vi "visualizer.vi"(11 "Name (\"\" to Use UUID)":string="ui") -> ()   [LabVIEW 2025]
uses:
  acccbc90-5136-4eb0-8ada-bd77d99bf855.vi
  <userlib>/_NEVSTOP/Communicable State Machine(CSM)/AdvanceAPI/CSM - Revert Arguments-Safe String.vi
  <userlib>/_NEVSTOP/Communicable State Machine(CSM)/AdvanceAPI/CSM - Make String Arguments Safe.vi
  <userlib>/_NEVSTOP/Communicable State Machine(CSM)/AdvanceAPI/CSM - Break Down Multiple States String.vi
  <userlib>/_NEVSTOP/Communicable State Machine(CSM)/AdvanceAPI/CSM - Compact Multiple States.vi
  <userlib>/_NEVSTOP/Communicable State Machine(CSM)/AdvanceAPI/CSM - Keywords.vi
  <userlib>/_NEVSTOP/Communicable State Machine(CSM)/_Shared/Trim Single-line Text.vi
  <userlib>/_NEVSTOP/Communicable State Machine(CSM)/addons/MassData-Parameter/_support/FGV-MassData(lvlibp).vi
  <userlib>/_NEVSTOP/Communicable State Machine(CSM)/_Polymophic/Build Asynchronous Message with Arguments.vi
  <userlib>/_NEVSTOP/Communicable State Machine(CSM)/Communicable State Machine.lvlib
panel:
  out "Error Occurred":errorcluster
  out "State History":string
  in  "Exit":bool
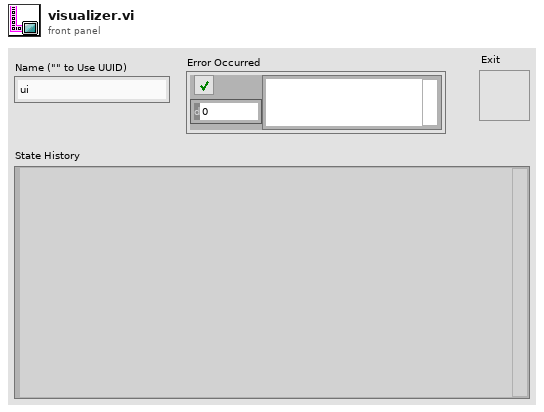
[diagram p1: front panel]
types:
  T1 = enum32{"Invalid", "Standard", "Closed", "Hidden", "Minimized", "Maximized"}
  T2 = enum32{"invalid app kind", "Development System", "Run Time System", "Student Edition", "Embedded LabVIEW", "Evaluation", "Custom"}
  T3 = typedef "Communicable State Machine.lvlib/_CSM_Response Source Message.ctl" = cluster{"‘State":string, "’Arguments":string, "’Error":errorcluster}
  T4 = cluster{"Current VI Reference":refnum<vi>, "Close Panel on Exit?":bool}
  T5 = cluster{"Core":cluster{"Current VI Reference":refnum<vi>, "Close Panel on Exit?":bool}, "rect":cluster{"left":i16, "top":i16, "right":i16, "bottom":i16}}
  T6 = cluster{"left":i16, "top":i16, "right":i16, "bottom":i16}
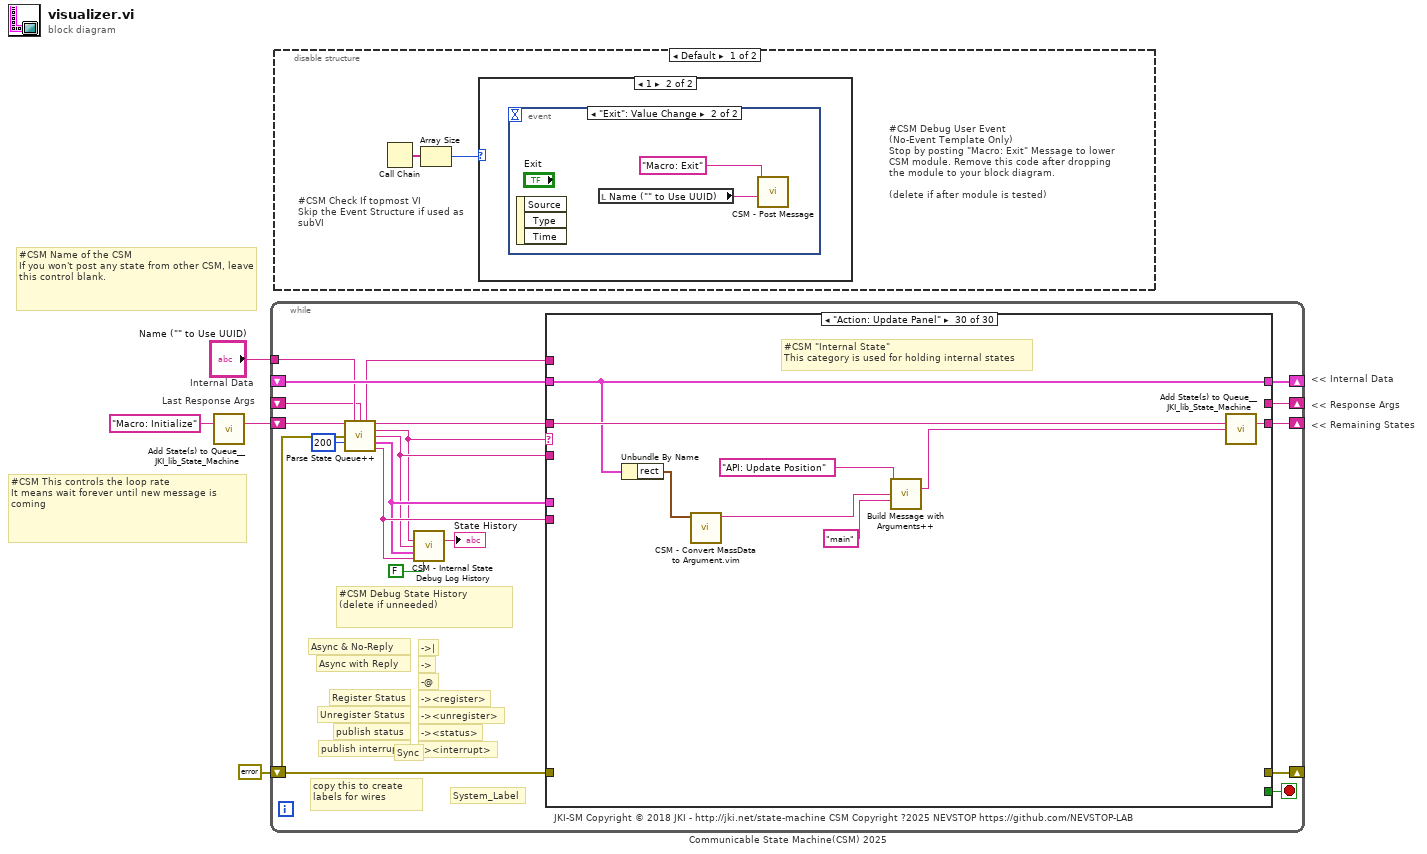
[diagram p0: block diagram]
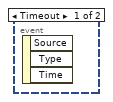
[diagram p3: hidden frame]
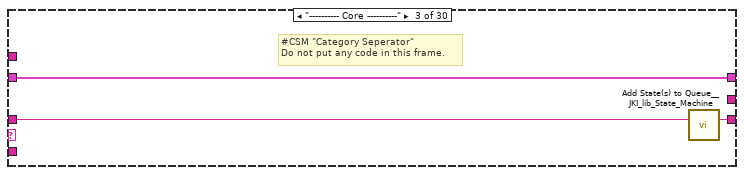
[diagram p7: hidden frame]
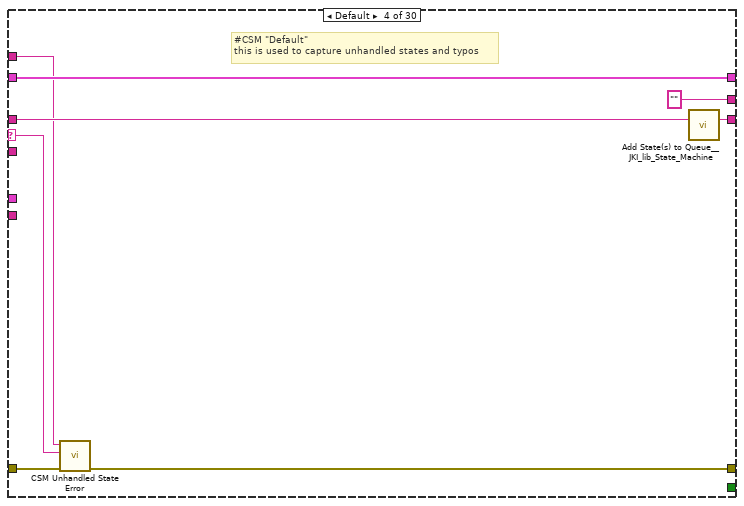
[diagram p8: hidden frame]
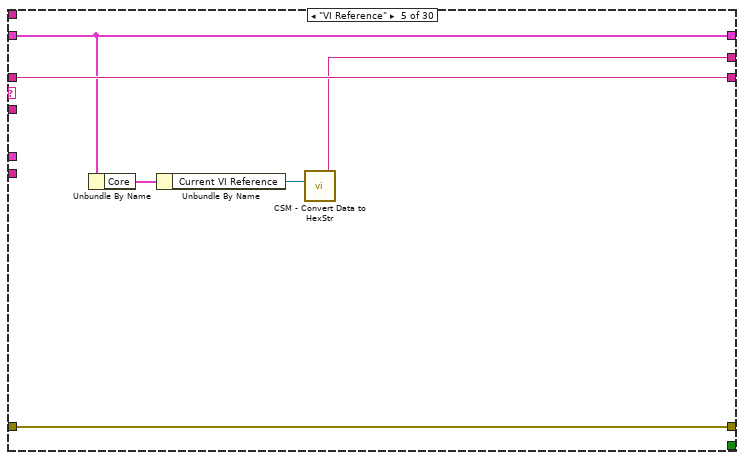
[diagram p9: hidden frame]
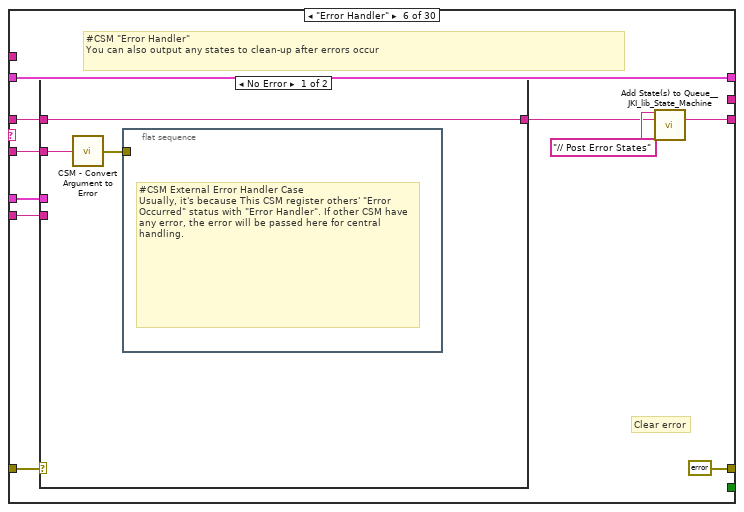
[diagram p10: hidden frame]
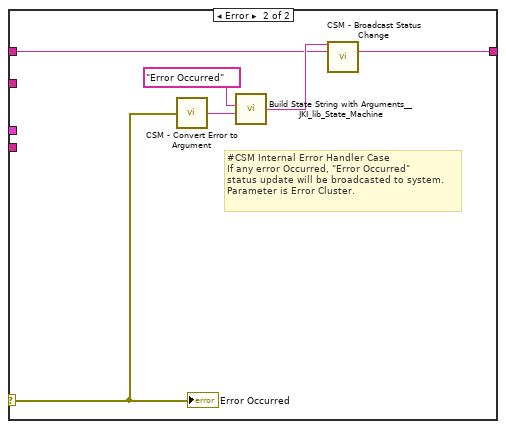
[diagram p11: hidden frame]
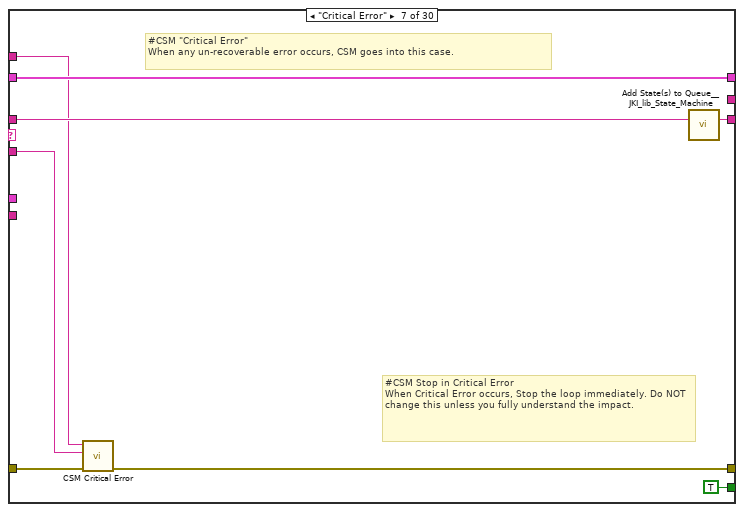
[diagram p12: hidden frame]
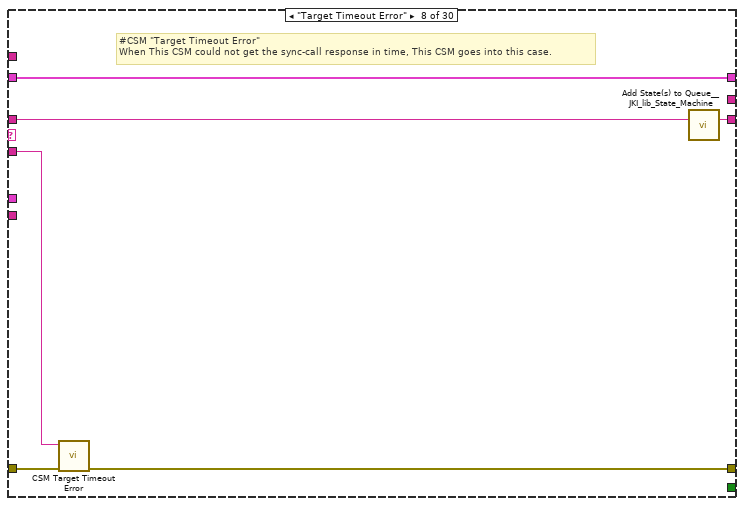
[diagram p13: hidden frame]
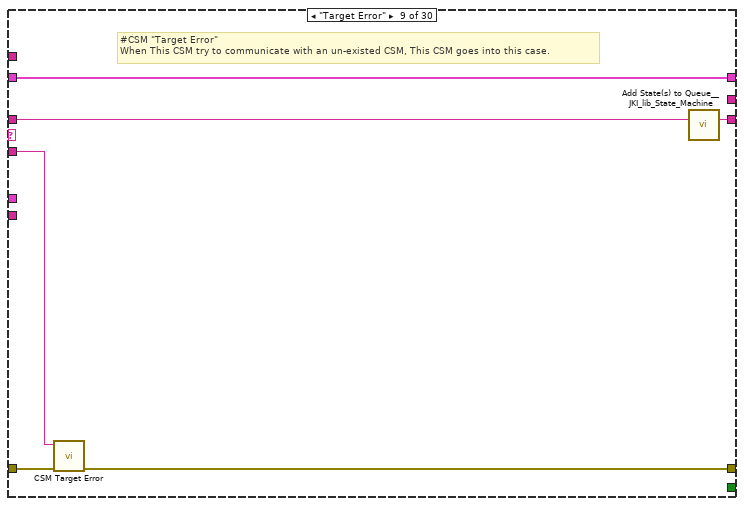
[diagram p14: hidden frame]
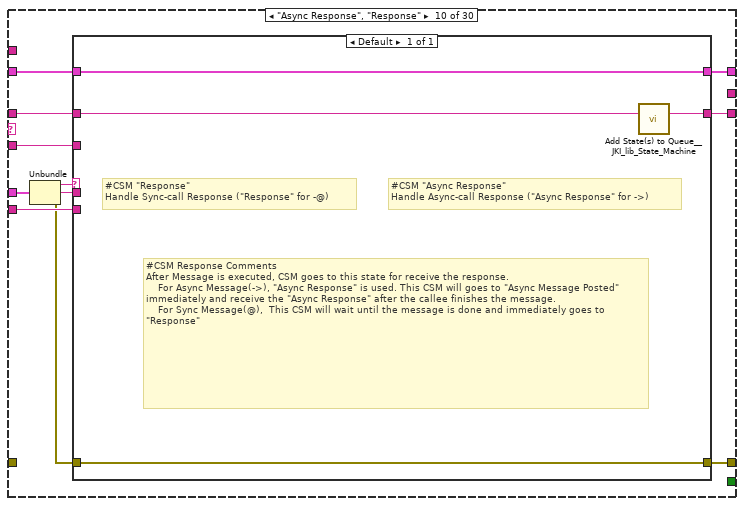
[diagram p15: hidden frame]
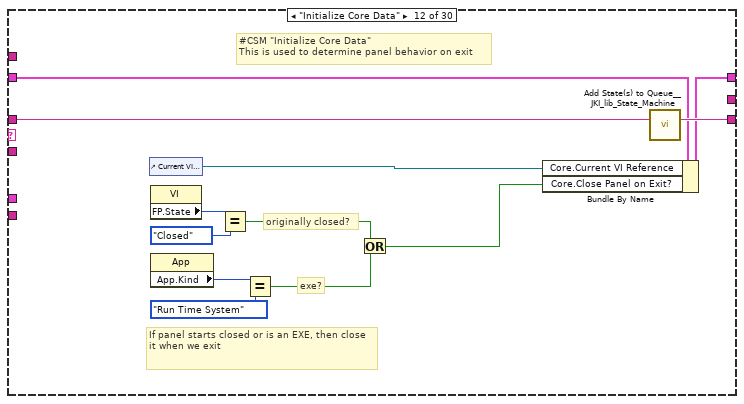
[diagram p17: hidden frame]
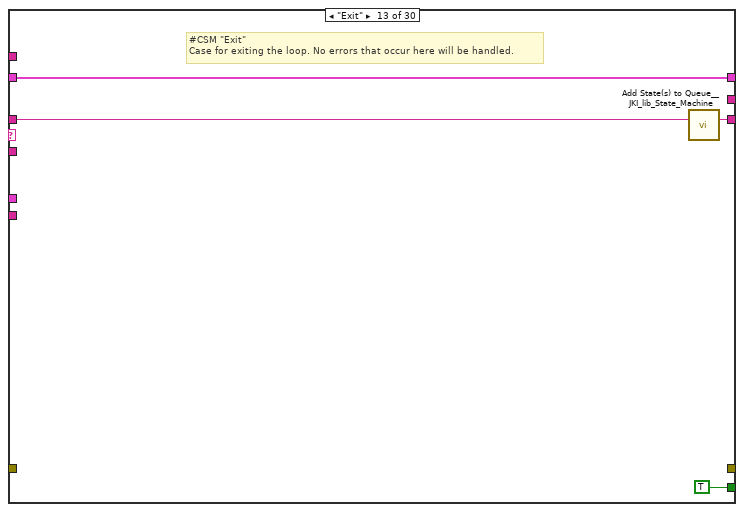
[diagram p18: hidden frame]
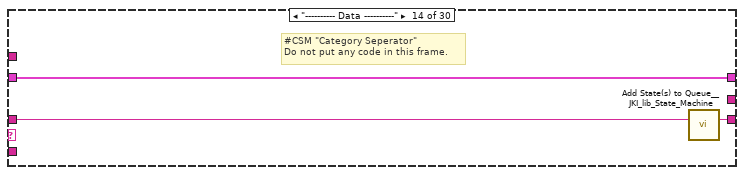
[diagram p19: hidden frame]
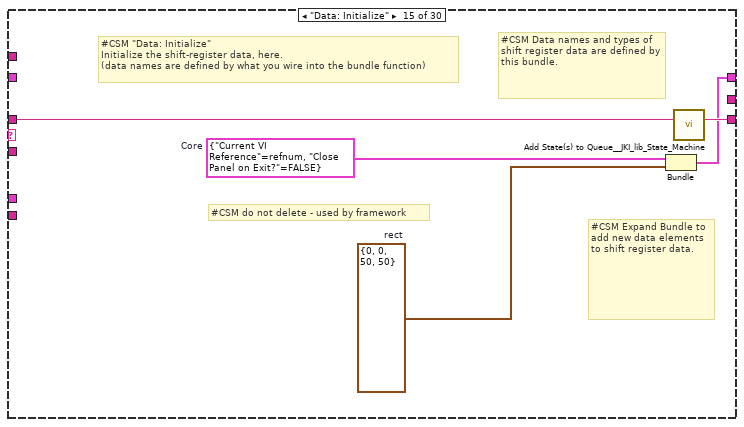
[diagram p20: hidden frame]
diagram:
  # "Last Response Args"
  # "Internal Data"
  # "#CSM Name of the CSM\nIf you won't post any state from other CSM, leave this control blank."
  # "#CSM This controls the loop rate\nIt means wait forever until new message is coming"
  # "<< Internal Data"
  # "<< Response Args"
  # "<< Remaining States"
  n1 = call <vilib>:"Add State(s) to Queue__JKI_lib_State_Machine.vi"("State(s) in (\"\")"="Macro: Initialize" ("Init State(\"Macro: Initialize\")")) -> ("States Out"=w1:string)  [unwired: 14 in]
  n2 = while "Communicable State Machine(CSM) 2025" {
    shift-right: [w18] -> _
    shift-left: _ -> [w17]
    shift-right: [w21] -> _
    shift-left: errorcluster {"status"=FALSE, "code"=0, "source"=""} ("error out") -> [w8]
    shift-right: [w20] -> _
    shift-left: w1 -> [w22]
    tunnel: "Name (\"\" to Use UUID)" -> [w15]
    shift-right: [w16] -> _
    shift-left: _ -> [w10]
    stop <- w19 stop-if-true
    # "#CSM Debug State History\n(delete if unneeded)"
    # "-><interrupt>"
    # "-><status>"
    # "-><unregister>"
    # "-><register>"
    # "-@"
    # "->"
    # "->|"
    # "publish interrupt"
    # "publish status"
    # "Unregister Status"
    # "Register Status"
    # "Sync"
    # "Async with Reply"
    # "Async & No-Reply"
    # "JKI-SM Copyright © 2018 JKI - http://jki.net/state-machine CSM Copyright ?2025 NEVSTOP https://github.com/NEVSTOP-LAB"
    # "copy this to create labels for wires"
    # "System_Label"
    n3 = call <userlib>:"Parse State Queue++.vi"("State Queue"=w22, "Name (\"\" to Use UUID)"=w15, "Response Arguments"=w10, "Previous Error"=w8, "Dequeue (1 ms)"=200) -> ("Name Used"=w9:string, "Remaining States"=w23:string, "Current State"=w11:string, "Arguments"=w12:string, "Additional Information"=w13:T3, "Source CSM"=w14:string)  [unwired: 5 in]
    n4 = call <userlib>:"CSM - Internal State Debug Log History.vi"("State"=w11, "Arguments (\"\")"=w12, ">> Response Source Message >>"=w13, "Source (\"\")"=w14, "Enable Periodic State Filter? (T)"=FALSE) -> ("Debug Log"=→"State History":string)  [unwired: 10 in]
    n5 = case shown="\"Action: Update Panel\"" w11 {
      selector: w11 -> [_ _ _ w34 _ _ _ _ _ _ _ _ _ _ _ _ _ _ _ _ _ _ _ _ _ _ _ _ _ _]
      tunnel: w23 -> [w24 w27 w30 w38 w43 w48 w71 w77 w83 w93 w100 w112 w116 w119 w124 w126 w132 w135 w139 w145 w147 w150 w153 w156 w166 w177 w188 w199 w203 w211]
      tunnel: w12 -> [_ _ _ _ _ w47 w67 w74 w80 w87 _ _ _ _ _ _ _ _ _ _ _ _ _ _ _ _ _ _ _ _]
      tunnel: w17 -> [w25 w26 w28 w36 w42 w53 w69 w75 w81 w91 w99 w106 w114 w117 _ w125 w127 w133 w137 w143 w146 w149 w152 w155 w160 w171 w182 w193 w201 w207]
      tunnel: [_ _ _ w31 w44 errorcluster {"status"=FALSE, "code"=0, "source"=""} ("error out") w64 w72 w78 w94 _ _ _ _ _ _ w128 _ _ _ w148 w151 w154 _ _ _ _ _ _ _] -> w21
      tunnel: w8 -> [_ _ _ w32 w44 w51 w65 w73 w79 _ _ _ _ _ _ _ w129 _ _ _ w148 w151 w154 _ _ _ _ _ _ _]
      tunnel: [w24 w27 w29 w37 w43 w49 w70 w76 w82 w92 w100 w111 w115 w118 w123 w126 w131 w134 w138 w144 w147 w150 w153 w156 w165 w176 w187 w198 w202 w210] -> w20
      tunnel: [_ _ _ _ _ _ TRUE _ _ _ _ _ TRUE _ _ _ _ _ _ _ _ _ _ _ _ _ _ _ _ _] -> w19
      tunnel: [w25 w26 w28 w36 w42 w53 w69 w75 w81 w90 w99 w110 w114 w117 w122 w125 w127 w133 w137 w143 w146 w149 w152 w155 w159 w170 w181 w192 w201 w207] -> w18
      tunnel: w14 -> [_ _ _ _ _ w46 _ _ _ w88 _ _ _ _ _ _ _ _ _ _ _ _ _ _ _ _ _ _ _ _]
      tunnel: w13 -> [_ _ _ _ _ w45 _ _ _ w89 _ _ _ _ _ _ _ _ _ _ _ _ _ _ _ _ _ _ _ _]
      tunnel: [_ _ _ "" w39 _ _ _ _ _ _ _ _ _ _ _ _ _ _ _ _ _ _ _ "Moved Up" ("HEX String (0-9,A-F)") "Moved Up" ("HEX String (0-9,A-F)") "Moved Up" ("HEX String (0-9,A-F)") "Moved Up" ("HEX String (0-9,A-F)") _ _] -> w16
      tunnel: w9 -> [_ _ _ w33 _ _ w66 _ _ _ _ _ _ _ _ _ _ _ _ _ _ _ _ _ _ _ _ _ _ _]
      frame "", "Idle" {
        # "#CSM \"Idle/Event Handler\"\nexecutes when the state queue is empty"
      }
      frame "CSM Documentation" {
        # "#CSM State Syntax\n\n// Comment line, all text to the right of “//” will be ignored\n// Local Message Example\nDoSth: DoA >> Arguments\n\n// Sync Call Example\nAPI: xxxx >> Arguments -@ TargetModule\n\n// Async Call Example\nAPI: xxxx >> Arguments -> TargetModule\n\n// Async Call without Reply Example\nAPI: xxxx >> Arguments ->| TargetModule\n\n// Broadcast normal status:\nStatus >> StatusArguments  -><status>\n\n// Broadcast Interrupt status:\nInterrupt >> StatusArguments  -><interrupt>\n\n// Register Source Module's status to Handler Module\nStatus@Source Module >> Handler Module@Handler Module -><register>\n\n// Unegister Source Module's status\nStatus@Source Module >> Handler Module -><unregister>"
        # "#CSM README FIRST\n\nCommunicable State Machine(CSM) is a LabVIEW application framework that builds upon JKI State Machine(JKISM). It follows the pattern of JKISM and extends the keywords to describe message communication between modules, including concepts such as Sync-Message, Async-Message, Subscription/Unsubscription of status - essential elements for creating reusable code modules. For more information, please visit the CSM wiki: https://nevstop-lab.github.io/CSM-Wiki/\n\nFor instructions on JKI State Machine, visit: \n    http://jki.net/state-machine/\nFor information about CSM, visit: \n    https://github.com/NEVSTOP-LAB"
        # "#CSM \"Documentation\"\nCase for holding CSM Documenation"
      }
      frame "---------- Core ----------" {
        # "#CSM \"Category Seperator\"\nDo not put any code in this frame."
        n6 = call <vilib>:"Add State(s) to Queue__JKI_lib_State_Machine.vi"("State(s) in (\"\")"=w30) -> ("States Out"=w29:string)  [unwired: 14 in]
      }
      frame Default {
        # "#CSM \"Default\"\nthis is used to capture unhandled states and typos"
        n7 = call <userlib>:"CSM Unhandled State Error.vi"("error in (no error)"=w32, "Undefined State"=w34, "CSM Name"=w33) -> ("error out"=w31:errorcluster)  [unwired: 8 in]
        n8 = call <vilib>:"Add State(s) to Queue__JKI_lib_State_Machine.vi"("State(s) in (\"\")"=w38) -> ("States Out"=w37:string)  [unwired: 14 in]
      }
      frame "VI Reference" {
        n9 = Unbundle By Name(w42) -> ("Core"=w41:T4)
        n10 = Unbundle By Name(w41) -> ("Current VI Reference"=w40:refnum<vi>)
        n11 = call <userlib>:"CSM - Convert Data to HexStr.vi"("Variant"=w40) -> ("HEX String (0-9,A-F)"=w39:string)  [unwired: 8 in]
      }
      frame "Error Handler" {
        # "#CSM \"Error Handler\"\nYou can also output any states to clean-up after errors occur"
        # "Clear error"
        n12 = case shown="No Error" w51 {
          selector: w51 -> [_ w58]
          tunnel: [w57 w60] -> w50
          tunnel: w48 -> [w57 w59]
          tunnel: w47 -> [w56 _]
          tunnel: w46 -> [_ _]
          tunnel: w45 -> [_ _]
          frame No Error {
            n13 = call <userlib>:"CSM - Convert Argument to Error.vi"("Argument"=w56) -> ("Error"=w55:errorcluster)  [unwired: 4 in]
            n14 = flat-sequence {
              tunnel: w55 -> [_]
              frame #0 {
                # "#CSM External Error Handler Case\nUsually, it's because This CSM register others' \"Error Occurred\" status with \"Error Handler\". If other CSM have any error, the error will be passed here for central handling."
              }
            }
          }
          frame Error {
            # "#CSM Internal Error Handler Case \nIf any error Occurred, \"Error Occurred\" \nstatus update will be broadcasted to system.\nParameter is Error Cluster."
            n15 = call <userlib>:"CSM - Convert Error to Argument.vi"("Error"=w58) -> ("Argument"=w62:string)  [unwired: 4 in]
            n16 = call <vilib>:"Build State String with Arguments__JKI_lib_State_Machine.vi"("Arguments (\"\")"=w62, "State"="Error Occurred" ("Status with Arguments")) -> ("State with Arguments"=w61:string)  [unwired: 4 in]
            n17 = call <userlib>:"CSM - Broadcast Status Change.vi"("Status With Arguments"=w61, "State Queue"=w59) -> ("Remaining States"=w60:string)  [unwired: 13 in]
            "Error Occurred" <- w58
          }
        }
        n18 = call <vilib>:"Add State(s) to Queue__JKI_lib_State_Machine.vi"("State(s) in Front (\"\")"="// Post Error States", "State(s) in (\"\")"=w50) -> ("States Out"=w49:string)  [unwired: 13 in]
      }
      frame "Critical Error" {
        # "#CSM \"Critical Error\"\nWhen any un-recoverable error occurs, CSM goes into this case."
        # "#CSM Stop in Critical Error\nWhen Critical Error occurs, Stop the loop immediately. Do NOT change this unless you fully understand the impact."
        n19 = call <userlib>:"CSM Critical Error.vi"("error in (no error)"=w65, "Arugments (As Reason)"=w67, "CSM Name"=w66) -> ("error out"=w64:errorcluster)  [unwired: 8 in]
        n20 = call <vilib>:"Add State(s) to Queue__JKI_lib_State_Machine.vi"("State(s) in (\"\")"=w71) -> ("States Out"=w70:string)  [unwired: 14 in]
      }
      frame "Target Timeout Error" {
        # "#CSM \"Target Timeout Error\"\nWhen This CSM could not get the sync-call response in time, This CSM goes into this case."
        n21 = call <userlib>:"CSM Target Timeout Error.vi"("error in (no error)"=w73, "Arguments (As CSM Name)"=w74) -> ("error out"=w72:errorcluster)  [unwired: 9 in]
        n22 = call <vilib>:"Add State(s) to Queue__JKI_lib_State_Machine.vi"("State(s) in (\"\")"=w77) -> ("States Out"=w76:string)  [unwired: 14 in]
      }
      frame "Target Error" {
        # "#CSM \"Target Error\"\nWhen This CSM try to communicate with an un-existed CSM, This CSM goes into this case."
        n23 = call <userlib>:"CSM Target Error.vi"("error in (no error)"=w79, "Arguments (As CSM Name)"=w80) -> ("error out"=w78:errorcluster)  [unwired: 9 in]
        n24 = call <vilib>:"Add State(s) to Queue__JKI_lib_State_Machine.vi"("State(s) in (\"\")"=w83) -> ("States Out"=w82:string)  [unwired: 14 in]
      }
      frame "Async Response", "Response" {
        n25 = Unbundle(w89) -> ("‘State"=w86:string, "’Arguments"=w85:string, "’Error"=w84:errorcluster)
        n26 = case shown="Default" w86 {
          tunnel: [w95] -> w92
          tunnel: w93 -> [w96]
          tunnel: [w98] -> w90
          tunnel: w91 -> [w98]
          tunnel: [w97] -> w94
          tunnel: w84 -> [w97]
          tunnel: w88 -> [_]
          tunnel: w87 -> [_]
          tunnel: w85 -> [_]
          frame Default {
            # "#CSM \"Async Response\"\nHandle Async-call Response (\"Async Response\" for ->)"
            # "#CSM \"Response\"\nHandle Sync-call Response (\"Response\" for -@)"
            # "#CSM Response Comments\nAfter Message is executed, CSM goes to this state for receive the response.\n    For Async Message(->), \"Async Response\" is used. This CSM will goes to \"Async Message Posted\" immediately and receive the \"Async Response\" after the callee finishes the message.\n    For Sync Message(@),  This CSM will wait until the message is done and immediately goes to \"Response\""
            n27 = call <vilib>:"Add State(s) to Queue__JKI_lib_State_Machine.vi"("State(s) in (\"\")"=w96) -> ("States Out"=w95:string)  [unwired: 14 in]
          }
        }
      }
      frame "Async Message Posted" {
        # "#CSM \"Async Message Posted\"\nAfter Async Message is posted (-> or ->| ), CSM goes to this state for post-action.\nYou can use Argument - State to tell which Async Message is called."
      }
      frame "Initialize Core Data" {
        # "#CSM \"Initialize Core Data\"\nThis is used to determine panel behavior on exit"
        # "originally closed?"
        # "exe?"
        # "If panel starts closed or is an EXE, then close it when we exit"
        n28 = control-ref of="Current VI Reference"() -> (w104:refnum<vi>)
        n29 = property class="VI"() -> ("FP.State"=w103:T1)  [unwired: 2 in, 2 out]
        n30 = property class="App"() -> ("App.Kind"=w109:T2)  [unwired: 2 in, 2 out]
        n31 = Equal?(x=w103, y=T1."Closed" ("Front Panel Window:State")) -> (x = y?=w101:bool)
        n32 = Equal?(x=w109, y=T2."Run Time System" ("Application:Kind")) -> (x = y?=w107:bool)
        n33 = Or(x=w101, y=w107) -> (x .or. y?=w105:bool)
        n34 = Bundle By Name(cluster=w106, "Core.Current VI Reference"=w104, "Core.Close Panel on Exit?"=w105) -> (w110:T5)
        n35 = call <vilib>:"Add State(s) to Queue__JKI_lib_State_Machine.vi"("State(s) in (\"\")"=w112) -> ("States Out"=w111:string)  [unwired: 14 in]
      }
      frame "Exit" {
        # "#CSM \"Exit\"\nCase for exiting the loop. No errors that occur here will be handled."
        n36 = call <vilib>:"Add State(s) to Queue__JKI_lib_State_Machine.vi"("State(s) in (\"\")"=w116) -> ("States Out"=w115:string)  [unwired: 14 in]
      }
      frame "---------- Data ----------" {
        # "#CSM \"Category Seperator\"\nDo not put any code in this frame."
        n37 = call <vilib>:"Add State(s) to Queue__JKI_lib_State_Machine.vi"("State(s) in (\"\")"=w119) -> ("States Out"=w118:string)  [unwired: 14 in]
      }
      frame "Data: Initialize" {
        w120 = T6 {"left"=0, "top"=0, "right"=50, "bottom"=50}  # rect
        w121 = T4 {"Current VI Reference"=refnum, "Close Panel on Exit?"=FALSE}  # Core
        # "#CSM \"Data: Initialize\"\nInitialize the shift-register data, here.\n(data names are defined by what you wire into the bundle function)"
        # "#CSM do not delete - used by framework"
        # "#CSM Expand Bundle to add new data elements to shift register data."
        # "#CSM Data names and types of shift register data are defined by this bundle."
        n38 = Bundle("Core"=w121, "rect"=w120) -> (w122:T5)  [unwired: 1 in]
        n39 = call <vilib>:"Add State(s) to Queue__JKI_lib_State_Machine.vi"("State(s) in (\"\")"=w124) -> ("States Out"=w123:string)  [unwired: 14 in]
      }
      frame "Data: Update Indicators" {
      }
      frame "Data: Cleanup" {
        # "#CSM \"Data: Cleanup\"\nCleanup any data and references, here.\n(this is called automatically, by the Macro: Exit)"
        n40 = Unbundle By Name(w127) -> ("Core.Current VI Reference"=w130:refnum<vi>)
        n41 = Close Reference(reference=w130, error in (no error)=w129) -> (error out=w128:errorcluster)
        n42 = call <vilib>:"Add State(s) to Queue__JKI_lib_State_Machine.vi"("State(s) in (\"\")"=w132) -> ("States Out"=w131:string)  [unwired: 14 in]
      }
      frame "---------- Macro ----------" {
        # "#CSM \"Category Seperator\"\nDo not put any code in this frame."
        n43 = call <vilib>:"Add State(s) to Queue__JKI_lib_State_Machine.vi"("State(s) in (\"\")"=w135) -> ("States Out"=w134:string)  [unwired: 14 in]
      }
      frame "Macro: Initialize" {
        # "#CSM \"Macro: Initialize\"\nInitialization Macro (This is called once, when the VI starts)"
        n44 = call <vilib>:"Add State(s) to Queue__JKI_lib_State_Machine.vi"("State(s) in Front (\"\")"="Initialize Core Data\nData: Initialize\nEvent: Register\nData: Update Indicators", "State(s) in (\"\")"=w139) -> ("States Out"=w138:string)  [unwired: 13 in]
      }
      frame "Macro: Exit" {
        # "#CSM \"Macro: Exit\"\nExit Macro (This is called once, when the VI exits)"
        n45 = call <vilib>:"Add State(s) to Queue__JKI_lib_State_Machine.vi"("State(s) in Front (\"\")"="//Exit Sub-Modules ", "State(s) at Back (\"\")"="Data: Cleanup\nExit") -> ("States Out"=w141:string)  [unwired: 13 in]
        n46 = call <vilib>:"Add State(s) to Queue__JKI_lib_State_Machine.vi"("State(s) in Front (\"\")"=w141, "State(s) in (\"\")"=w145) -> ("States Out"=w144:string)  [unwired: 13 in]
      }
      frame "---------- Event ----------" {
      }
      frame "Event: Register" {
      }
      frame "Event: Unregister" {
      }
      frame "---------- API ----------" {
        # "#CSM \"Category Seperator\"\nDo not put any code in this frame."
      }
      frame "API: Up" {
        w161 = i16 -20 ("y")
        # "#CSM API Example\nCopy/Rename this case for your own API"
        n47 = Unbundle By Name(w160) -> ("rect.top"=w163:i16, "rect.bottom"=w162:i16)
        n48 = Add(x=w162, y=w161) -> (x+y=w157:i16)
        n49 = Add(x=w163, y=w161) -> (x+y=w158:i16)
        n50 = Bundle By Name(cluster=w160, "rect.top"=w158, "rect.bottom"=w157) -> (w159:T5)
        n51 = call <vilib>:"Add State(s) to Queue__JKI_lib_State_Machine.vi"("State(s) in (\"\")"=w166, "State(s) at Back (\"\")"="Action: Update Panel" ("State(s) at Back (\"\")")) -> ("States Out"=w165:string)  [unwired: 13 in]
      }
      frame "API: Down" {
        w172 = i16 20 ("y")
        # "#CSM API Example\nCopy/Rename this case for your own API"
        n52 = Unbundle By Name(w171) -> ("rect.top"=w174:i16, "rect.bottom"=w173:i16)
        n53 = Add(x=w173, y=w172) -> (x+y=w168:i16)
        n54 = Add(x=w174, y=w172) -> (x+y=w169:i16)
        n55 = Bundle By Name(cluster=w171, "rect.top"=w169, "rect.bottom"=w168) -> (w170:T5)
        n56 = call <vilib>:"Add State(s) to Queue__JKI_lib_State_Machine.vi"("State(s) in (\"\")"=w177, "State(s) at Back (\"\")"="Action: Update Panel" ("State(s) at Back (\"\")")) -> ("States Out"=w176:string)  [unwired: 13 in]
      }
      frame "API: Left" {
        w183 = i16 -20 ("y")
        # "#CSM API Example\nCopy/Rename this case for your own API"
        n57 = Unbundle By Name(w182) -> ("rect.left"=w185:i16, "rect.right"=w184:i16)
        n58 = Add(x=w184, y=w183) -> (x+y=w179:i16)
        n59 = Add(x=w185, y=w183) -> (x+y=w180:i16)
        n60 = Bundle By Name(cluster=w182, "rect.left"=w180, "rect.right"=w179) -> (w181:T5)
        n61 = call <vilib>:"Add State(s) to Queue__JKI_lib_State_Machine.vi"("State(s) in (\"\")"=w188, "State(s) at Back (\"\")"="Action: Update Panel" ("State(s) at Back (\"\")")) -> ("States Out"=w187:string)  [unwired: 13 in]
      }
      frame "API: Right" {
        w194 = i16 20 ("y")
        # "#CSM API Example\nCopy/Rename this case for your own API"
        n62 = Unbundle By Name(w193) -> ("rect.left"=w196:i16, "rect.right"=w195:i16)
        n63 = Add(x=w195, y=w194) -> (x+y=w190:i16)
        n64 = Add(x=w196, y=w194) -> (x+y=w191:i16)
        n65 = Bundle By Name(cluster=w193, "rect.left"=w191, "rect.right"=w190) -> (w192:T5)
        n66 = call <vilib>:"Add State(s) to Queue__JKI_lib_State_Machine.vi"("State(s) in (\"\")"=w199, "State(s) at Back (\"\")"="Action: Update Panel" ("State(s) at Back (\"\")")) -> ("States Out"=w198:string)  [unwired: 13 in]
      }
      frame "---------- Action ----------" {
        # "#CSM \"Category Seperator\"\nDo not put any code in this frame."
        n67 = call <vilib>:"Add State(s) to Queue__JKI_lib_State_Machine.vi"("State(s) in (\"\")"=w203) -> ("States Out"=w202:string)  [unwired: 14 in]
      }
      frame "Action: Update Panel" {
        # "#CSM \"Internal State\"\nThis category is used for holding internal states"
        n68 = Unbundle By Name(w207) -> ("rect"=w206:T6)
        n69 = call "CSM - Convert MassData to Argument.vim"("Data"=w206) -> ("MassData Argument"=w205:string)  [unwired: 7 in, 1 out]
        n70 = call-poly <userlib>:"Build Message with Arguments++.vi"("State With Arguments"="API: Update Position", "Arguments (\"\")"=w205, "Target Module (\"\")"="main" ("Target Module (\"\")")) -> ("CSM Message String"=w204:string)  [unwired: 12 in]
        n71 = call <vilib>:"Add State(s) to Queue__JKI_lib_State_Machine.vi"("State(s) in (\"\")"=w211, "State(s) at Back (\"\")"=w204) -> ("States Out"=w210:string)  [unwired: 13 in]
      }
    }
  }
  n72 = disable-structure shown="Default" {
    frame condition #0 (active) {
      # "#CSM Check If topmost VI\nSkip the Event Structure if used as subVI"
      # "#CSM Debug User Event\n(No-Event Template Only)\nStop by posting \"Macro: Exit\" Message to lower CSM module. Remove this code after dropping the module to your block diagram. \n\n(delete if after module is tested)"
      n73 = Call Chain() -> (call chain=w213:string[])
      n74 = Array Size(array=w213) -> (size(s)=w212:i32)
      n75 = case shown="1" w212 {
        frame Default {
        }
        frame 1 {
          n76 = event shown="[1] \"Exit\": Value Change" {
            selector: _ -> [_ _]
            dyn-events: _ -> [_ _]
            timeout: _ -> [_ _]
            event Timeout {
              n77 = event-data() -> ()  [unwired: 1 in, 3 out]
            }
            event "Exit": Value Change {
              n78 = event-data() -> ()  [unwired: 1 in, 3 out]
              n79 = local read "Name (\"\" to Use UUID)"() -> (w215:string)
              n80 = call <userlib>:"CSM - Post Message.vi"("Target Module"=w215, "State"="Macro: Exit" ("States")) -> ()  [unwired: 9 in, 1 out]
            }
          }
        }
      }
    }
    frame condition #1 {
    }
  }
